vi "JSON to SHW file.vi"(8 "error in (no error)":errorcluster, 10 "Capabilities JSON In":string, 11 "device":string) -> (0 "error out":errorcluster, 2 "SLSC Switch Info":refnum<class "Relay.lvclass">[](array[class]), 3 "SHW Path Out":path)   [LabVIEW 2015, in "SLSC Switch.lvlib" / "SLSC Switch.lvclass"]
uses:
  SLSC Switch.lvclass
  Relay/Relay.lvclass
  Controls/JSON.Relay.ctl
  Controls/JSON.RelaySLSCAction.ctl
  Relay/Property.ctl
  Relay/Command.ctl
  <vilib>/Utility/config.llb/Write Key (I32).vi
  <vilib>/Utility/config.llb/NI_LVConfig.lvlib
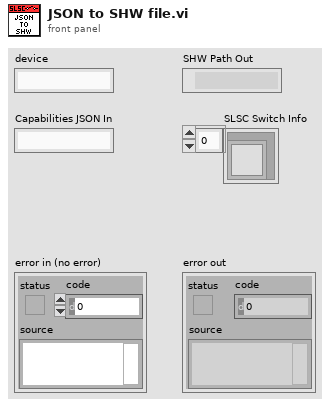
[diagram p1: front panel]
types:
  T1 = typedef "SLSC Switch.lvlib/SLSC Switch.lvclass/JSON.Relay.ctl" = cluster{"name":string, "actions":T2[]}
  T2 = typedef "SLSC Switch.lvlib/SLSC Switch.lvclass/JSON.RelaySLSCAction.ctl" = cluster{"type":string, "resource":string, "value":string}
  T3 = typedef "SLSC Switch.lvlib/Relay.lvclass/Property.ctl" = cluster{"resource name":string, "property":refnum<k21>}
  T4 = typedef "SLSC Switch.lvlib/Relay.lvclass/Command.ctl" = cluster{"resource name":string, "command":refnum<k21>}
  T5 = typedef "NI_LVConfig.lvlib/Config Data RefNum.ctl" = refnum<k1>
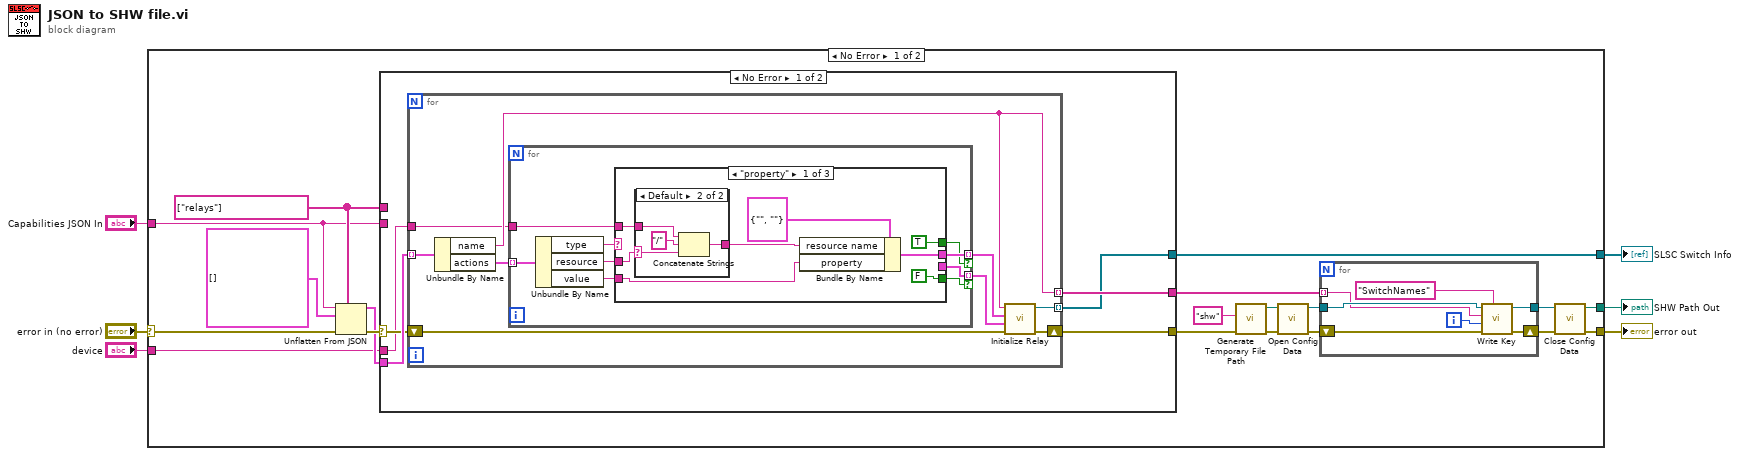
[diagram p0: block diagram]
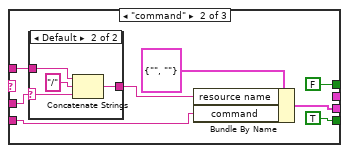
[diagram p3: hidden frame]
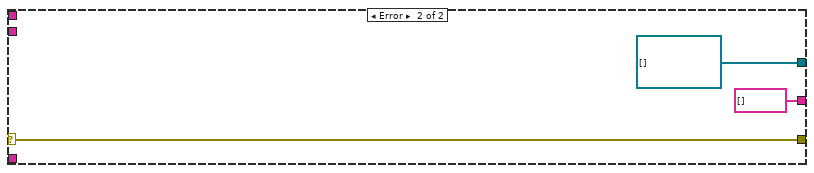
[diagram p6: hidden frame]
diagram:
  n1 = case shown="No Error" "error in (no error)" {
    selector: "error in (no error)" -> [w25 w86]
    tunnel: [w18 w86] -> w5
    tunnel: "Capabilities JSON In" -> [w10 _]
    tunnel: [w16 _] -> w3
    tunnel: "device" -> [w8 _]
    tunnel: [w13 _] -> w1
    frame No Error {
      w11 = string[] ["relays"] ("path")
      n2 = Unflatten From JSON(path=w11, JSON string=w10, type and defaults=T1[] [] ("Array"), error in (no error)=w25) -> (value=w14:T1[], error out=w15:errorcluster)  [unwired: 3 in]
      n3 = case shown="No Error" w15 {
        selector: w15 -> [w28 w78]
        tunnel: w14 -> [w31 _]
        tunnel: [w30 string[] []] -> w9
        tunnel: [w29 refnum<class "Relay.lvclass">[] []] -> w13
        tunnel: [w27 w78] -> w12
        tunnel: w11 -> [_ _]
        tunnel: w10 -> [_ _]
        tunnel: w8 -> [w26 _]
        frame No Error {
          n4 = for {
            tunnel: w31 -> [w37] mode=indexing
            tunnel: [w35] -> w30 mode=indexing
            tunnel: [w40] -> w29 mode=indexing
            shift-right: [w38] -> w27
            shift-left: w28 -> [w39]
            tunnel: w26 -> [w32]
            n5 = Unbundle By Name(w37) -> ("name"=w35:string, "actions"=w36:T2[])
            n6 = for {
              tunnel: w36 -> [w49] mode=indexing
              tunnel: [w45] -> w34 mode=indexing if=w43
              tunnel: [w44] -> w33 mode=indexing if=w42
              tunnel: w32 -> [w41]
              n7 = Unbundle By Name(w49) -> ("type"=w48:string, "resource"=w47:string, "value"=w46:string)
              n8 = case shown="\"property\"" w48 {
                tunnel: w47 -> [w52 w63 _]
                tunnel: w46 -> [w56 w70 _]
                tunnel: [w55 _ _] -> w45
                tunnel: [TRUE FALSE _] -> w43
                tunnel: [_ w67 _] -> w44
                tunnel: [FALSE TRUE _] -> w42
                tunnel: w41 -> [w51 w65 _]
                frame "property" {
                  n9 = case shown="Default" w52 {
                    selector: w52 -> [_ w59]
                    tunnel: w51 -> [w58 w61]
                    tunnel: [w58 w60] -> w50
                    frame "device" {
                    }
                    frame Default {
                      n10 = Concatenate Strings(w61, "/" ("string"), w59) -> (w60:string)
                    }
                  }
                  n11 = Bundle By Name(cluster=T3 {"resource name"="", "property"=""} ("Property"), "resource name"=w50, "property"=w56) -> (w55:T3)
                }
                frame "command" {
                  n12 = case shown="Default" w63 {
                    selector: w63 -> [_ w72]
                    tunnel: w65 -> [w71 w74]
                    tunnel: [w71 w73] -> w64
                    frame "device" {
                    }
                    frame Default {
                      n13 = Concatenate Strings(w74, "/" ("string"), w72) -> (w73:string)
                    }
                  }
                  n14 = Bundle By Name(cluster=T4 {"resource name"="", "command"=""} ("Command"), "resource name"=w64, "command"=w70) -> (w67:T4)
                }
                frame Default {
                }
              }
            }
            n15 = call "Initialize Relay.vi"("error in (no error)"=w39, "Commands"=w33, "Properties"=w34, "name"=w35) -> ("error out"=w38:errorcluster, "Relay out"=w40:refnum<class "Relay.lvclass">)  [unwired: 6 in]
          }
        }
        frame Error {
        }
      }
      n16 = call <vilib>:"Generate Temporary File Path.vi"("error in (no error)"=w12, "Temporary File Extension (tmp)"="shw") -> ("error out"=w23:errorcluster, "Unique Temporary File Path"=w17:path)  [unwired: 8 in]
      n17 = call <vilib>:"Open Config Data.vi"("error in (no error)"=w23, "configuration file path"=w17) -> ("error out"=w21:errorcluster, "refnum"=w22:T5)  [unwired: 7 in, 1 out]
      n18 = for {
        tunnel: w22 -> [w85]
        tunnel: [w84] -> w19
        shift-right: [w82] -> w20
        shift-left: w21 -> [w83]
        tunnel: w9 -> [w79] mode=indexing
        i -> [w80]
        n19 = call-poly <vilib>:"Write Key.vi"("section"="SwitchNames", "error in (no error)"=w83, "value"=w80, "key"=w79, "refnum"=w85) -> ("error out"=w82:errorcluster, "refnum out"=w84:T5)  [unwired: 4 in, 1 out]
      }
      n20 = call <vilib>:"Close Config Data.vi"("error in (no error)"=w20, "refnum"=w19) -> ("error out"=w18:errorcluster, "file path"=w16:path)  [unwired: 8 in]
    }
    frame Error {
    }
  }
  "error out" <- w5
  "SHW Path Out" <- w3
  "SLSC Switch Info" <- w1
